vi "get error start of range.vi"() -> (3 "Start of Error Range":i32)   [LabVIEW 2013, in "Linux Errno.lvlib"]
uses:
  Linux Errno.lvlib
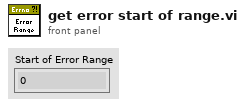
[diagram p1: front panel]
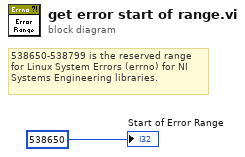
[diagram p0: block diagram]
diagram:
  # "538650-538799 is the reserved range for Linux System Errors (errno) for NI Systems Engineering libraries."
  "Start of Error Range" <- 538650
